vi "Action.vi"(8 "error in (no error)":errorcluster, 10 "Actor in":refnum<class "Tamagotchi Basic Actor.lvclass">, 11 "Message in":refnum<class "Message.lvclass">) -> (0 "error out":errorcluster, 2 "Actor out":refnum<class "Tamagotchi Basic Actor.lvclass">, 3 "Message out":refnum<class "Message.lvclass">)   [LabVIEW 2026, in "Message.lvclass"]
uses:
  Message.lvclass
  Tamagotchi Basic Actor/Tamagotchi Basic Actor.lvclass
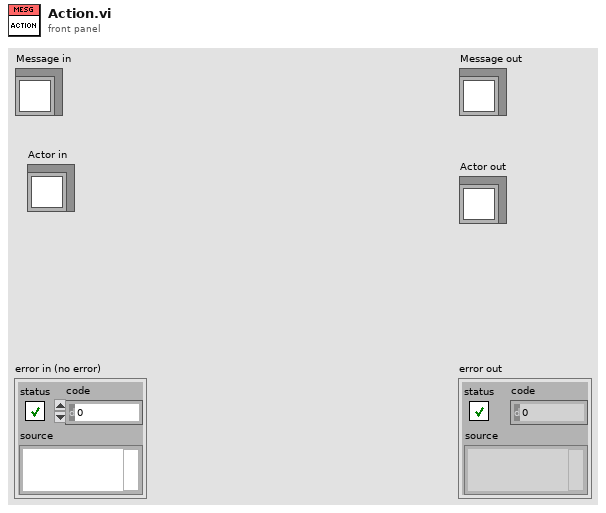
[diagram p1: front panel]
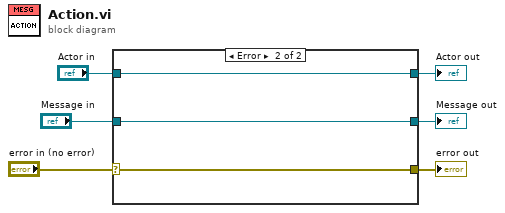
[diagram p0: block diagram]
diagram:
  n1 = case shown="Error" "error in (no error)" {
    selector: "error in (no error)" -> [w8 w12]
    tunnel: [w8 w12] -> w5
    tunnel: [w9 w11] -> w3
    tunnel: "Message in" -> [w9 w11]
    tunnel: [w7 w10] -> w2
    tunnel: "Actor in" -> [w7 w10]
    frame No Error {
      # "Wire the error cluster across even in the \"No Error\"\ncase so that warnings get propagated."
    }
    frame Error {
    }
  }
  "error out" <- w5
  "Message out" <- w3
  "Actor out" <- w2
